vi "CC Observation List to Table.vi"(8 "error in (no error)":errorcluster, 11 "Observation List":T2[](array[typedef])) -> (0 "error out":errorcluster, 1 "Screen Ready Table":string[][](array[string]), 2 "Status":T1[](array[typedef]), 3 "File Ready Table":string[][](array[string]))   [LabVIEW 2024]
uses:
  typedefs/CC cluster Observation.ctl
  Observation Queue/CC enum Observation Status.ctl
  Telescope/CC cluster Telescope Offsets.ctl
  typedefs/CC cluster Observation Dither Options.ctl
  typedefs/CC enum Dither Selection.ctl
panel:
  out "Header":string[](array[string])
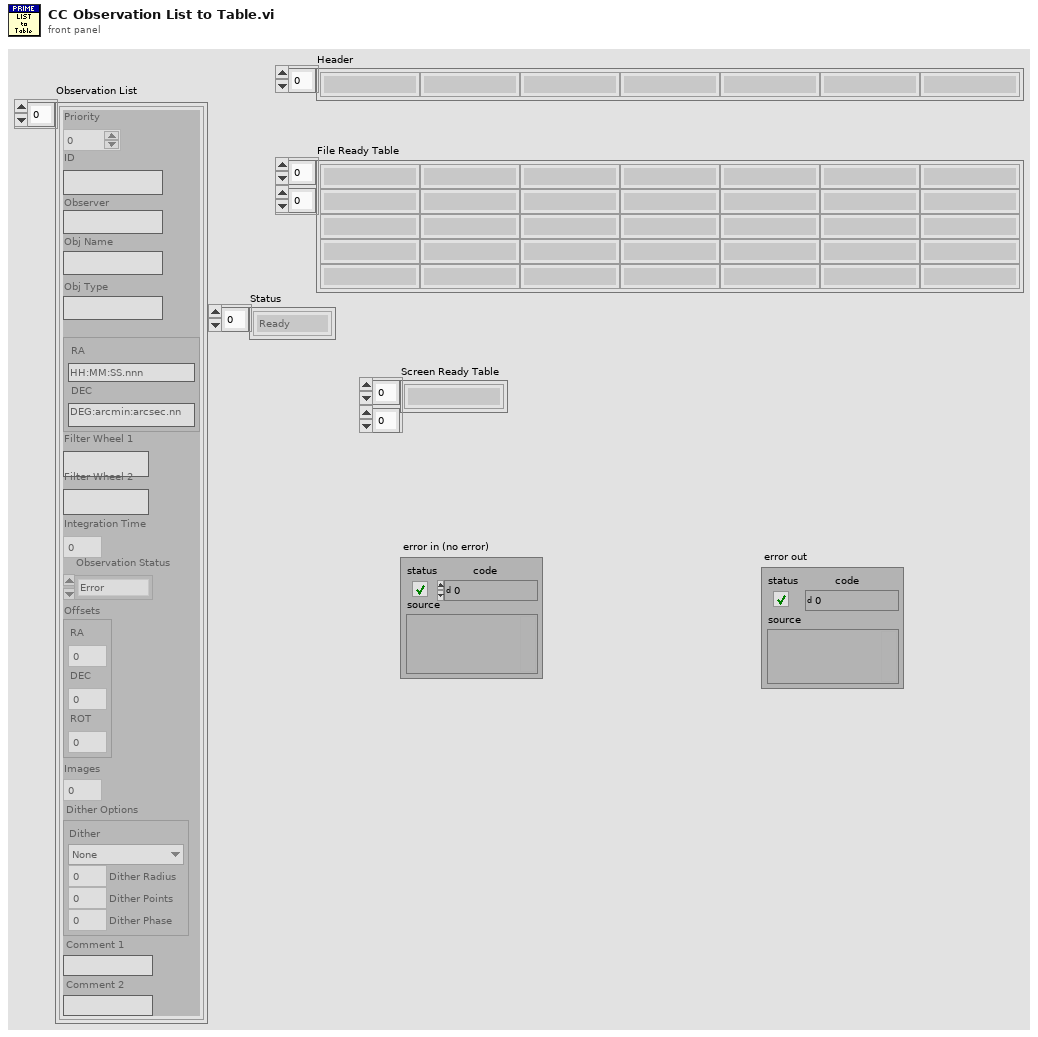
[diagram p1: front panel]
types:
  T1 = typedef "CC enum Observation Status.ctl" = enum16{"Ready", "Running", "Done", "Error"}
  T2 = typedef "CC cluster Observation.ctl" = cluster{"Priority":i32, "ID":string, "Observer":string, "Obj Name":string, "Obj Type":string, "RA and DEC String":cluster{"RA":string, "DEC":string}, "Filter Wheel 1":string, "Filter Wheel 2":string, "Integration Time":dbl, "Observation Status":T1, "Offsets":T3, "Images":i32, "Dither Options":T4, "Comment 1":string, "Comment 2":string}
  T3 = typedef "CC cluster Telescope Offsets.ctl" = cluster{"RA":dbl, "DEC":dbl, "ROT":dbl}
  T4 = typedef "CC cluster Observation Dither Options.ctl" = cluster{"Dither":T5, "Dither Radius":dbl, "Dither Points":i32, "Dither Phase":dbl}
  T5 = typedef "CC enum Dither Selection.ctl" = enum16{"None", "Circle", "Random"}
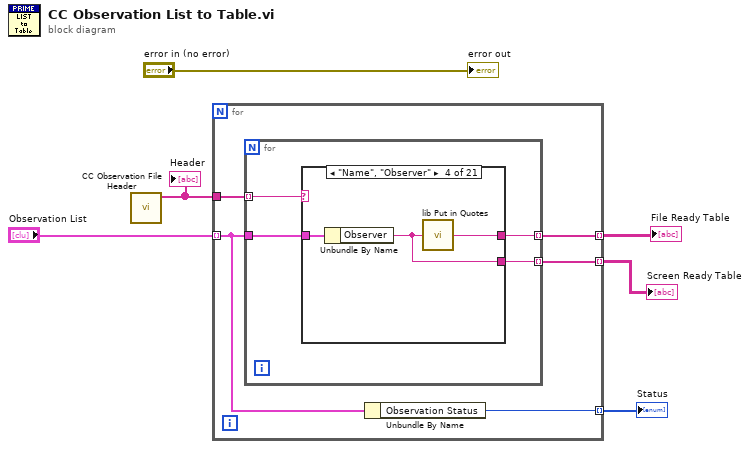
[diagram p0: block diagram]
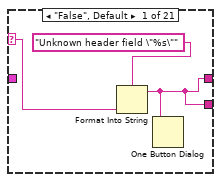
[diagram p2: hidden frame]
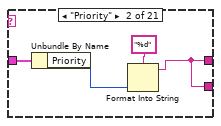
[diagram p3: hidden frame]
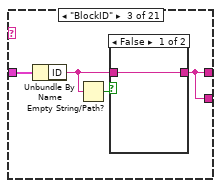
[diagram p4: hidden frame]
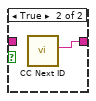
[diagram p5: hidden frame]
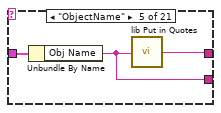
[diagram p6: hidden frame]
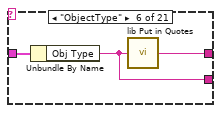
[diagram p7: hidden frame]
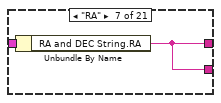
[diagram p8: hidden frame]
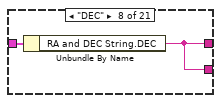
[diagram p9: hidden frame]
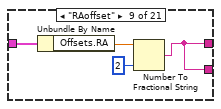
[diagram p10: hidden frame]
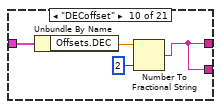
[diagram p11: hidden frame]
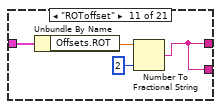
[diagram p12: hidden frame]
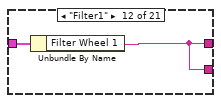
[diagram p13: hidden frame]
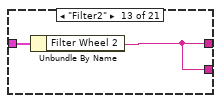
[diagram p14: hidden frame]
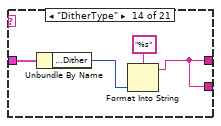
[diagram p15: hidden frame]
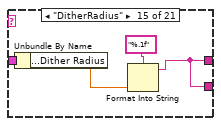
[diagram p16: hidden frame]
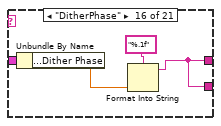
[diagram p17: hidden frame]
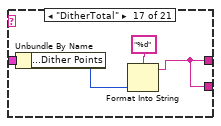
[diagram p18: hidden frame]
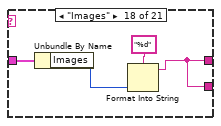
[diagram p19: hidden frame]
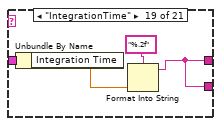
[diagram p20: hidden frame]
diagram:
  n1 = call "CC Observation File Header.vi"() -> ("Header"=w5:string[])  [unwired: 10 in, 1 out]
  "Header" <- w5
  n2 = for {
    tunnel: w5 -> [w11]
    tunnel: "Observation List" -> [w9] mode=indexing
    tunnel: [w10] -> w3 mode=indexing
    tunnel: [w8] -> w4 mode=indexing
    tunnel: [w7] -> w1 mode=indexing
    n3 = for {
      tunnel: w11 -> [w15] mode=indexing
      tunnel: w9 -> [w14]
      tunnel: [w13] -> w10 mode=indexing
      tunnel: [w12] -> w7 mode=indexing
      n4 = case shown="\"Name\", \"Observer\"" w15 {
        selector: w15 -> [w17 _ _ _ _ _ _ _ _ _ _ _ _ _ _ _ _ _ _ _ _]
        tunnel: w14 -> [_ w22 w26 w31 w34 w37 w39 w41 w45 w49 w53 w55 w57 w61 w65 w69 w73 w77 w81 w84 w87]
        tunnel: [w16 w19 w23 w30 w33 w36 w38 w40 w42 w46 w50 w54 w56 w58 w62 w66 w70 w74 w78 w82 w85] -> w13
        tunnel: [w16 w19 w23 w29 w32 w35 w38 w40 w42 w46 w50 w54 w56 w58 w62 w66 w70 w74 w78 w82 w85] -> w12
        frame "False", Default {
          n5 = Format Into String(format string="Unknown header field \"%s\"" ("Filter Wheel 2"), w17) -> (resulting string=w16:string)  [unwired: 2 in, 1 out]
          n6 = One Button Dialog(message=w16) -> ()  [unwired: 1 in, 1 out]
        }
        frame "Priority" {
          n7 = Unbundle By Name(w22) -> ("Priority"=w20:i32)
          n8 = Format Into String(format string="%d", w20) -> (resulting string=w19:string)  [unwired: 2 in, 1 out]
        }
        frame "BlockID" {
          n9 = Unbundle By Name(w26) -> ("ID"=w24:string)
          n10 = Empty String/Path?(string/path=w24) -> (empty?=w25:bool)
          n11 = case shown="False" w25 {
            tunnel: [w27 w28] -> w23
            tunnel: w24 -> [w27 _]
            frame False {
            }
            frame True {
              n12 = call "CC Next ID.vi"() -> ("BlockID string"=w28:string)  [unwired: 9 in, 2 out]
            }
          }
        }
        frame "Name", "Observer" {
          n13 = Unbundle By Name(w31) -> ("Observer"=w29:string)
          n14 = call "lib Put in Quotes.vi"("String"=w29) -> ("Quoted String"=w30:string)  [unwired: 4 in]
        }
        frame "ObjectName" {
          n15 = Unbundle By Name(w34) -> ("Obj Name"=w32:string)
          n16 = call "lib Put in Quotes.vi"("String"=w32) -> ("Quoted String"=w33:string)  [unwired: 4 in]
        }
        frame "ObjectType" {
          n17 = Unbundle By Name(w37) -> ("Obj Type"=w35:string)
          n18 = call "lib Put in Quotes.vi"("String"=w35) -> ("Quoted String"=w36:string)  [unwired: 4 in]
        }
        frame "RA" {
          n19 = Unbundle By Name(w39) -> ("RA and DEC String.RA"=w38:string)
        }
        frame "DEC" {
          n20 = Unbundle By Name(w41) -> ("RA and DEC String.DEC"=w40:string)
        }
        frame "RAoffset" {
          n21 = Unbundle By Name(w45) -> ("Offsets.RA"=w44:dbl)
          n22 = Number To Fractional String(number=w44, precision (6)=i16 2) -> (F-format string=w42:string)  [unwired: 2 in]
        }
        frame "DECoffset" {
          n23 = Unbundle By Name(w49) -> ("Offsets.DEC"=w48:dbl)
          n24 = Number To Fractional String(number=w48, precision (6)=i16 2) -> (F-format string=w46:string)  [unwired: 2 in]
        }
        frame "ROToffset" {
          n25 = Unbundle By Name(w53) -> ("Offsets.ROT"=w52:dbl)
          n26 = Number To Fractional String(number=w52, precision (6)=i16 2) -> (F-format string=w50:string)  [unwired: 2 in]
        }
        frame "Filter1" {
          n27 = Unbundle By Name(w55) -> ("Filter Wheel 1"=w54:string)
        }
        frame "Filter2" {
          n28 = Unbundle By Name(w57) -> ("Filter Wheel 2"=w56:string)
        }
        frame "DitherType" {
          n29 = Unbundle By Name(w61) -> ("Dither Options.Dither"=w59:T5)
          n30 = Format Into String(format string="%s", w59) -> (resulting string=w58:string)  [unwired: 2 in, 1 out]
        }
        frame "DitherRadius" {
          n31 = Unbundle By Name(w65) -> ("Dither Options.Dither Radius"=w63:dbl)
          n32 = Format Into String(format string="%.1f", w63) -> (resulting string=w62:string)  [unwired: 2 in, 1 out]
        }
        frame "DitherPhase" {
          n33 = Unbundle By Name(w69) -> ("Dither Options.Dither Phase"=w67:dbl)
          n34 = Format Into String(format string="%.1f", w67) -> (resulting string=w66:string)  [unwired: 2 in, 1 out]
        }
        frame "DitherTotal" {
          n35 = Unbundle By Name(w73) -> ("Dither Options.Dither Points"=w71:i32)
          n36 = Format Into String(format string="%d", w71) -> (resulting string=w70:string)  [unwired: 2 in, 1 out]
        }
        frame "Images" {
          n37 = Unbundle By Name(w77) -> ("Images"=w75:i32)
          n38 = Format Into String(format string="%d", w75) -> (resulting string=w74:string)  [unwired: 2 in, 1 out]
        }
        frame "IntegrationTime" {
          n39 = Unbundle By Name(w81) -> ("Integration Time"=w79:dbl)
          n40 = Format Into String(format string="%.2f", w79) -> (resulting string=w78:string)  [unwired: 2 in, 1 out]
        }
        frame "Comment1" {
          n41 = Unbundle By Name(w84) -> ("Comment 1"=w83:string)
          n42 = call "lib Put in Quotes.vi"("String"=w83) -> ("Quoted String"=w82:string)  [unwired: 4 in]
        }
        frame "Comment2" {
          n43 = Unbundle By Name(w87) -> ("Comment 2"=w86:string)
          n44 = call "lib Put in Quotes.vi"("String"=w86) -> ("Quoted String"=w85:string)  [unwired: 4 in]
        }
      }
    }
    n45 = Unbundle By Name(w9) -> ("Observation Status"=w8:T1)
  }
  "File Ready Table" <- w3
  "Status" <- w4
  "Screen Ready Table" <- w1
  "error out" <- "error in (no error)"
